vi "Test Apply Bounds.vi"() -> ()   [LabVIEW 2011]
uses:
  Vec3d Class.lvclass
panel:
  out "Bounded":cluster{"X":dbl, "Y":dbl, "Z":dbl}
  in  "Bounds":cluster{"X":dbl, "Y":dbl, "Z":dbl}
  in  "Vector":cluster{"X":dbl, "Y":dbl, "Z":dbl}
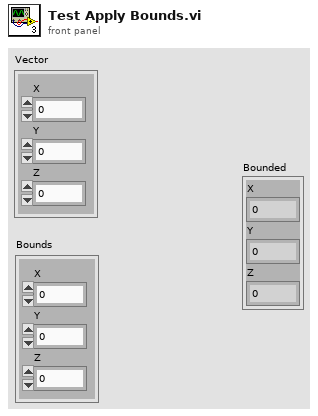
[diagram p1: front panel]
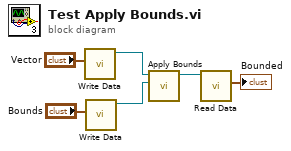
[diagram p0: block diagram]
diagram:
  n1 = call "Write Data.vi"("Data"="Vector") -> ("Vec3d Class out"=w4:refnum<class "Vec3d Class.lvclass">)  [unwired: 9 in, 1 out]
  n2 = call "Write Data.vi"("Data"="Bounds") -> ("Vec3d Class out"=w3:refnum<class "Vec3d Class.lvclass">)  [unwired: 9 in, 1 out]
  n3 = call "Apply Bounds.vi"("Bounds"=w3, "Vec3d in"=w4) -> ("Vec3d out"=w2:refnum<class "Vec3d Class.lvclass">)  [unwired: 8 in, 1 out]
  n4 = call-dynamic "Read Data.vi"("Vec3d Class in"=w2) -> ("Data"=→"Bounded":cluster{"X":dbl, "Y":dbl, "Z":dbl})  [unwired: 8 in, 2 out]
